vi "Trim string both ends to just decimals.vi"(8 "error in (no error)":errorcluster, 11 "string":string) -> (0 "error out":errorcluster, 3 "String out":string)   [LabVIEW 2013]
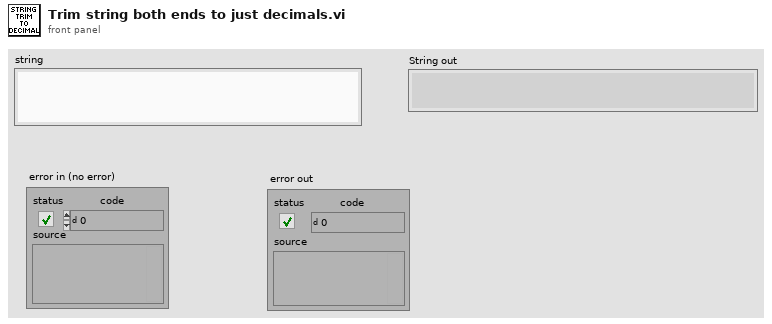
[diagram p1: front panel]
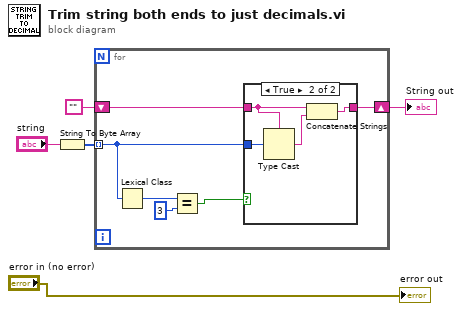
[diagram p0: block diagram]
diagram:
  n1 = String To Byte Array(string="string") -> (unsigned byte array=w4:u8[])
  n2 = for {
    tunnel: w4 -> [w8] mode=indexing
    shift-right: [w9] -> w2
    shift-left: "" -> [w10]
    n3 = Lexical Class(1:w8) -> (0:w7:i16)
    n4 = Equal?(x=w7, y=i16 3) -> (x = y?=w6:bool)
    n5 = case shown="True" w6 {
      tunnel: w10 -> [w12 w14]
      tunnel: [w12 w16] -> w9
      tunnel: w8 -> [_ w15]
      frame False {
      }
      frame True {
        n6 = Type Cast(type=w14, x=w15) -> (*(type *) &x=w13:string)
        n7 = Concatenate Strings(w14, w13) -> (w16:string)
      }
    }
  }
  "String out" <- w2
  "error out" <- "error in (no error)"
